vi "Aero_tunnel_monitor_on_OGI.vi"() -> ()   [LabVIEW 2014]
uses:
  Controls/Post_Process.ctl
  <vilib>/Platform/TimedLoop/XDataNode/timing_clust.ctl
  <vilib>/Platform/TimedLoop/XDataNode/nitl_modes.ctl
  <vilib>/Platform/TimedLoop/XDataNode/wakeup.ctl
  ADAM Client/Sub VIs/ADAM Controls/Update_scan_value.ctl
  Globals/Meas_global.vi
  <vilib>/Platform/TimedLoop/XDataNode/XDataNode.xnode
  <vilib>/Platform/TimedLoop/XDataNode/XDNodeRunTimeDep.lvlib
panel:
  in  "Use Polynomial for Ratio":bool
  in  "Manual Ratio":dbl=1.02
  in  "Display Graph?":bool
  in  "Menu Ring":u16(ring) items=["Lift", "Pitch", "Drag", "Side", "Yaw", "Roll"]
  in  "Samples":i32=1000
  out "Waveform Chart":dbl[](graph)
  in  "Output Roll":bool
  out "Roll":string="0.0 Nm"
  in  "Output Yaw":bool
  out "Yaw":string="0.0 Nm"
  in  "Output Pitch":bool
  out "Pitch":string="0.0 Nm"
  in  "Output SF":bool
  out "SF":string="0.0 N"
  in  "Output Drag":bool
  out "Drag":string="0.0 N"
  in  "Output Lift":bool
  out "Lift":string="0.0 N"
  in  "Balance Safety limits":T1(array[cluster])=[{"Max +ve Range"=80, "Max -ve Range"=80, "Axis"="Lift"}, {"Max +ve Range"=80, "Max -ve Range"=80, "Axis"="Pitch"}, {"Max +ve Range"=80, "Max -ve Range"=80, "Axis"="Drag"}, {"Max +ve Range"=80, "Max -ve Range"=80, "Axis"="Side-Force"}, {"Max +ve Range"=99, "Max -ve Range"=99, "Axis"="Yaw"}, {"Max +ve Range"=80, "Max -ve Range"=80, "Axis"="Roll"}] {"Max -ve Range" min=0 max=125; "Max +ve Range" min=0 max=125}
  out "Monitor Speed (Hz)":dbl
  out "Belt slip warning":bool
  out "Road Status":string="???"
  in  "GotoYaw":bool
  in  "NewYawPos":dbl
  out "YAW POSITION":dbl
  out "Required WindSpeedRatio":dbl
  out "ROAD SPEED m/s":dbl
  in  "BL Fan1":i32
  in  "BL Fan2":i32
  in  "Stop drive":bool
  in  "Start Drive":bool
  in  "Synch to Wind":bool
  out "Road Info":string="???"
  in  "stop":bool
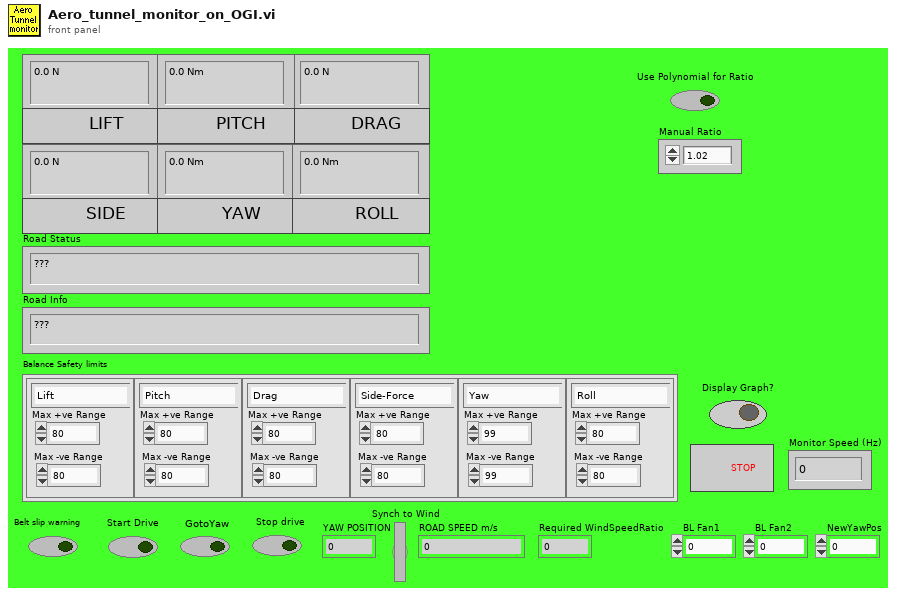
[diagram p1: front panel]
types:
  T1 = cluster{"Max +ve Range":i32, "Max -ve Range":i32, "Axis":string}[]
  T2 = typedef "Post_Process.ctl" = enum16{"Take New Data", "Post Process Raw Data File"}
  T3 = typedef "XDNodeRunTimeDep.lvlib/timing_clust.ctl" = cluster{"Expected End [f-1]":u64, "Actual End [f-1]":u64, "Finished Late? [f-1]":bool, "Expected End [i-1]":u64, "Actual End [i-1]":u64, "Finished Late? [i-1]":bool, "Expected Start [i]":u64, "Actual Start [i]":u64, "Expected Start [f]":u64, "Actual Start [f]":u64, "Source Name":string, "Structure Name":string, "Period":i64, "Deadline":i64, "Offset":i64, "Start":i64, "Priority":i32, "Timeout":i32, "Mode":T4, "Wakeup Reason":T5, "Error":errorcluster, "Source Type":string, "Secondary Source Type":string, "Global End Time":u64, "Global Start Time":u64, "Frame Duration":u64, "Iteration Duration":u64, "Assigned CPU":i32, "I/O Scan Engine Mode":u32}
  T4 = typedef "XDNodeRunTimeDep.lvlib/nitl_modes.ctl" = enum32{"No Change", "Process missed periods, maintain original phase", "Discard missed periods, maintain original phase", "Process missed periods, ignore original phase", "Discard missed periods, ignore original phase"}
  T5 = typedef "XDNodeRunTimeDep.lvlib/wakeup.ctl" = enum32{"Normal", "Aborted", "Asynchronous wakeup", "Timing source error", "Timed loop error", "Timeout"}
  T6 = typedef "Update_scan_value.ctl" = cluster{"Channel Name":string, "New Value":dbl}
  T7 = cluster{"Max +ve Range":i32, "Max -ve Range":i32, "Axis":string}
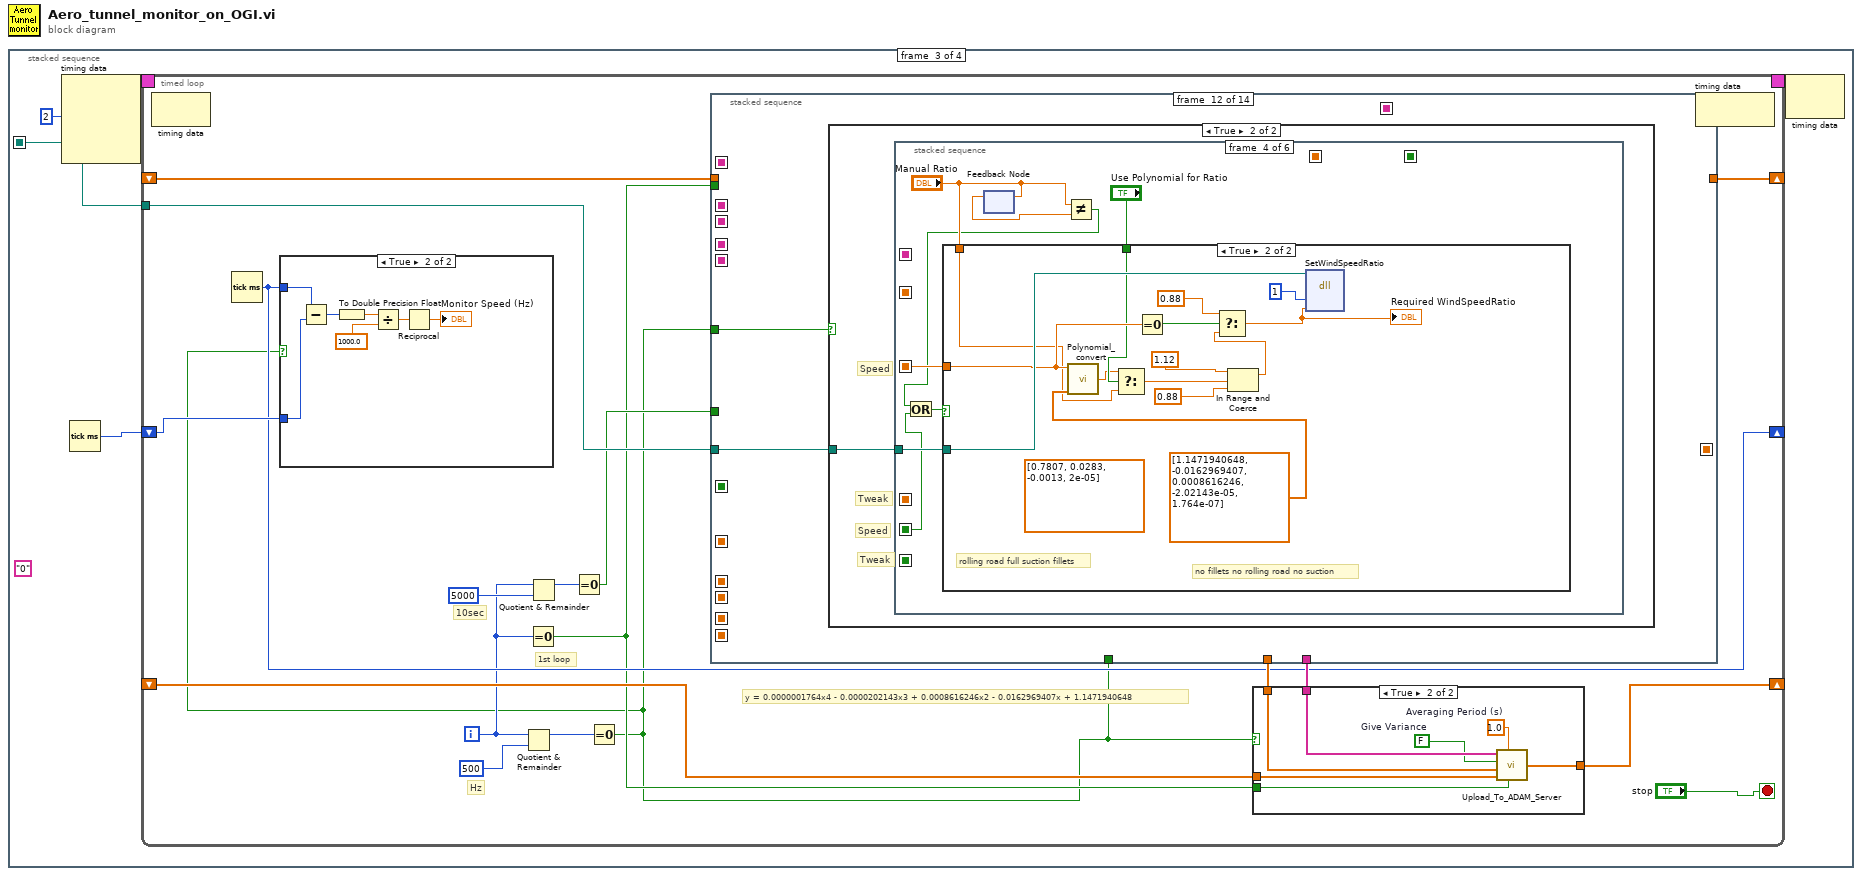
[diagram p0: block diagram]
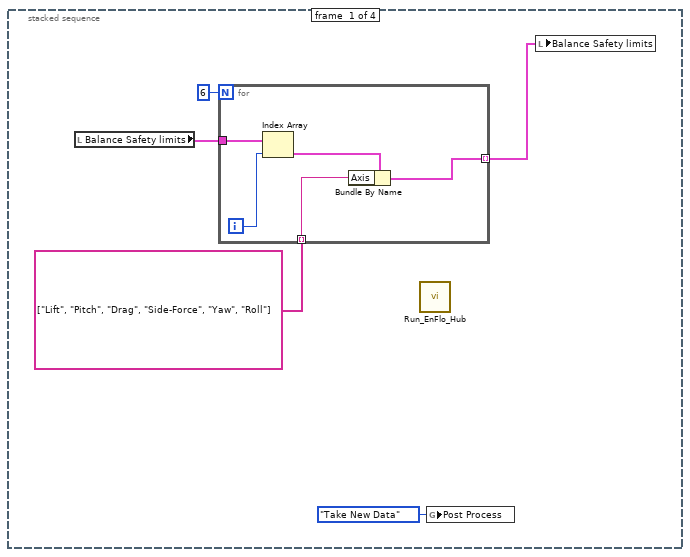
[diagram p2: hidden frame]
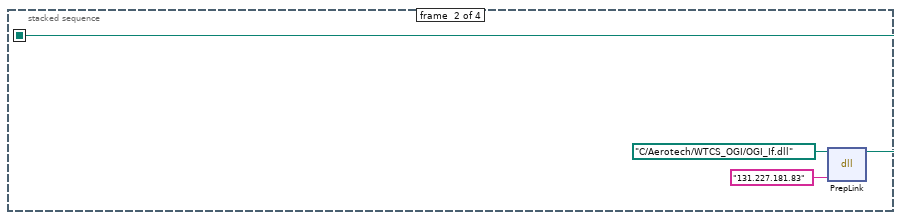
[diagram p3: hidden frame]
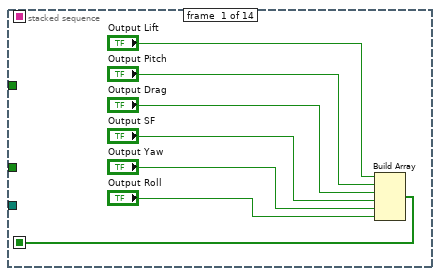
[diagram p6: hidden frame]
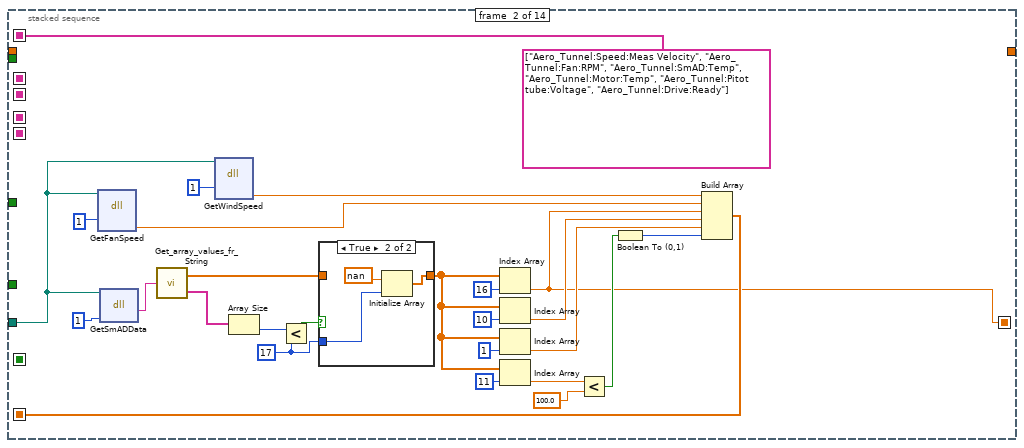
[diagram p7: hidden frame]
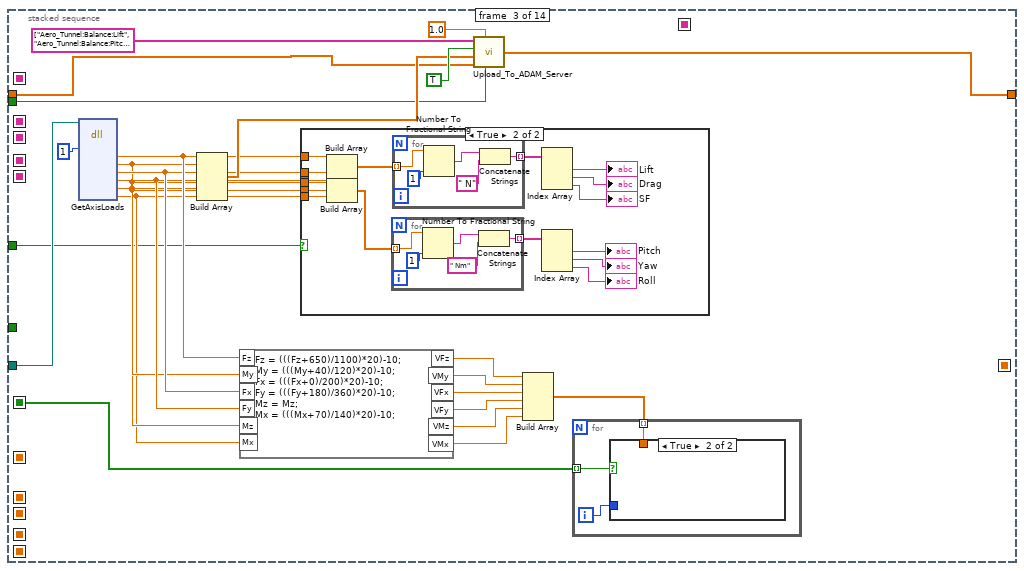
[diagram p9: hidden frame]
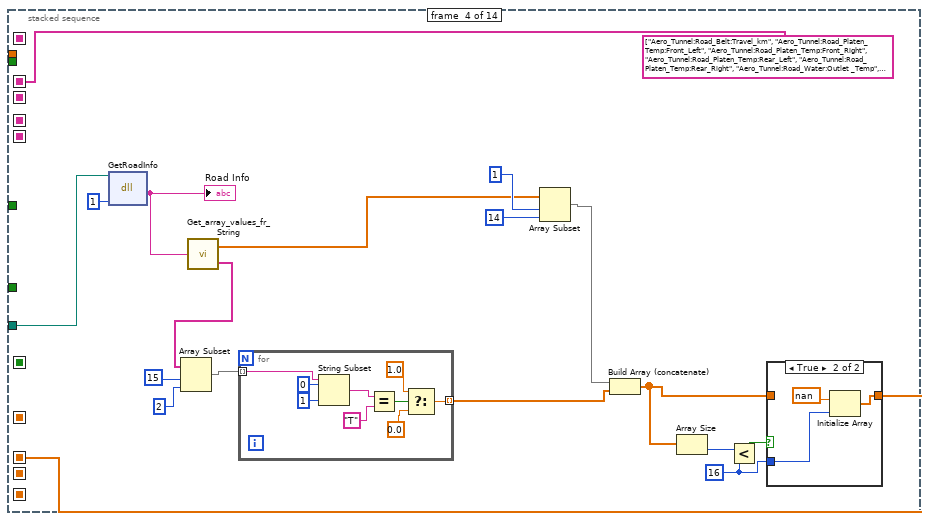
[diagram p12: hidden frame]
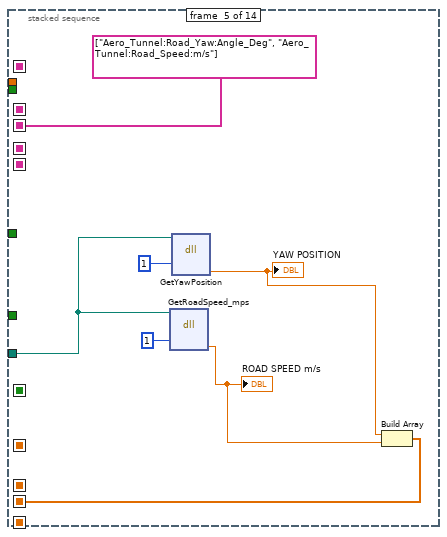
[diagram p14: hidden frame]
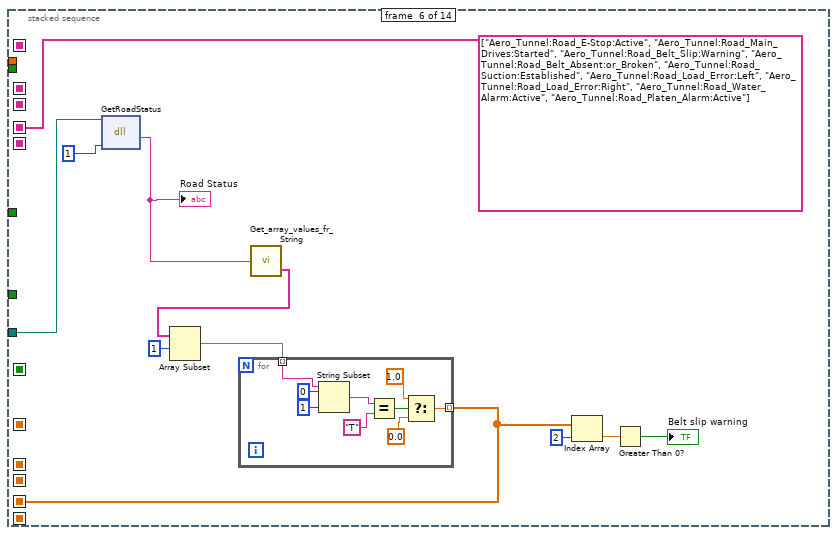
[diagram p15: hidden frame]
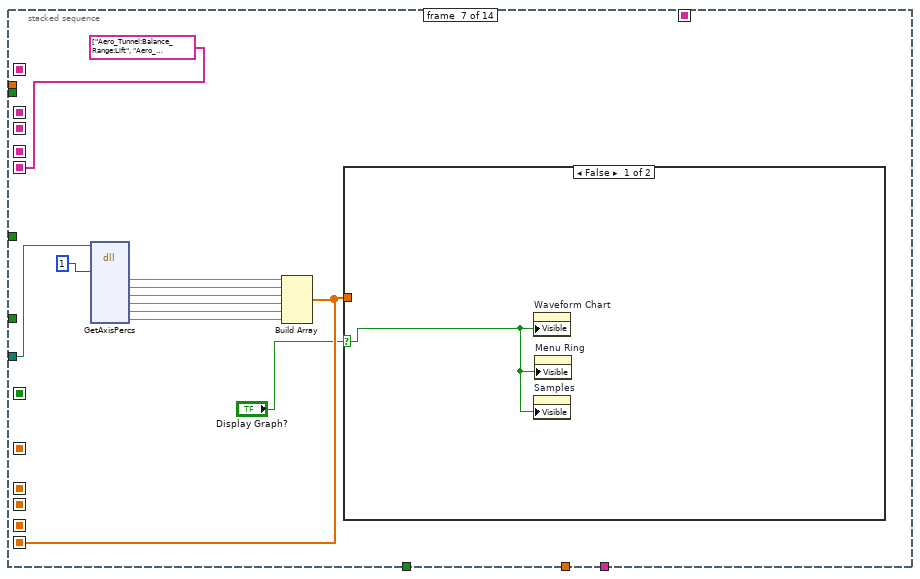
[diagram p16: hidden frame]
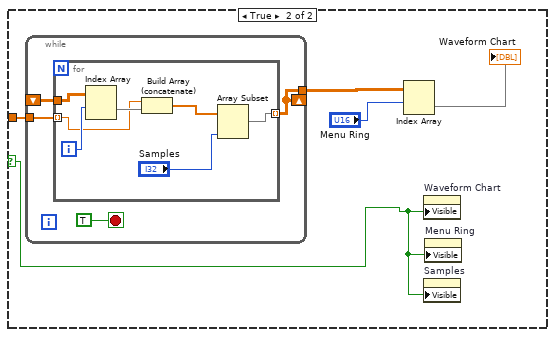
[diagram p17: hidden frame]
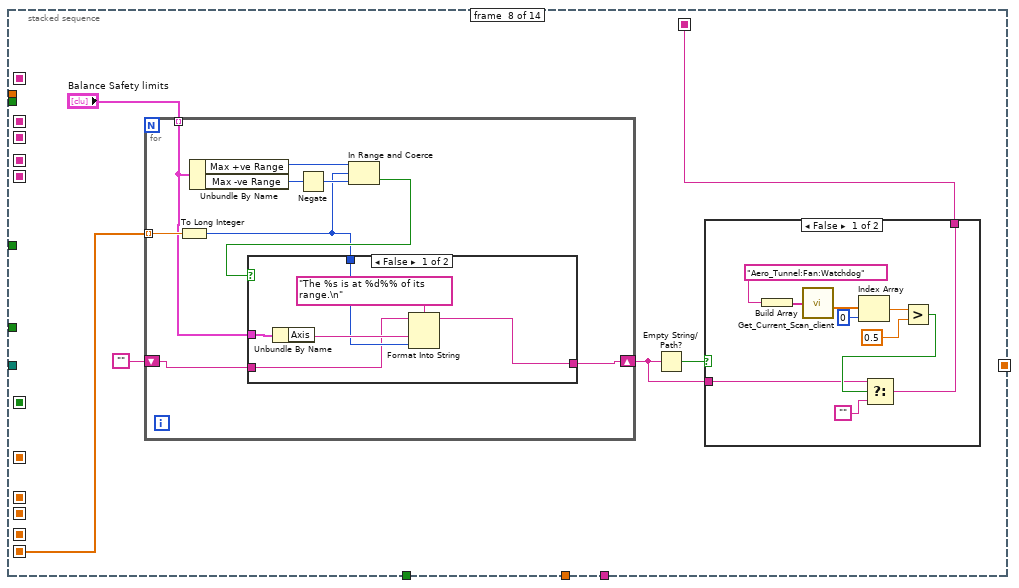
[diagram p18: hidden frame]
diagram:
  n1 = stacked-sequence {
    seq-local: [_ w11 _ _] -> [_ _ w18 w513]
    frame #0 {
      n2 = local read "Balance Safety limits"() -> (w4:T1)
      n3 = for {
        N: 6 -> [_]
        tunnel: w4 -> [w10]
        tunnel: [w7] -> w3 mode=indexing
        tunnel: string[] ["Lift", "Pitch", "Drag", "Side-Force", "Yaw", "Roll"] ("Channel Names") -> [w6] mode=indexing
        i -> [w9]
        n4 = Index Array(array=w10, index=w9) -> (element=w8:T7)
        n5 = Bundle By Name(cluster=w8, "Axis"=w6) -> (w7:T7)
      }
      n6 = call "Run_EnFlo_Hub.vi"() -> ()  [unwired: 8 in]
      n7 = global write "Meas_global.vi" "Post Process"(Post_Process."Take New Data" ("Post Process")) -> ()
      n8 = local write "Balance Safety limits"(w3) -> ()
    }
    frame #1 {
      n9 = dll-call lib="C:/Aerotech/Drivers/OGI_IF.dll" fn="PrepLink"(path in=path "C:/Aerotech/WTCS_OGI/OGI_If.dll", "IPAddress"="131.227.181.83") -> (path out=w11:path)  [unwired: 2 in, 3 out]
    }
    frame #2 {
      (unwired) "0" ("Channels")
      n10 = node-c288(i64 2 ("Period")) -> (w16:T3)  [unwired: 3 in]
      n11 = Tick Count (ms)() -> (millisecond timer value=w17:u32)
      n12 = timed-loop {
        shift-right: [w36] -> _
        shift-left: _ -> [w34]
        tunnel: w18 -> [w32]
        shift-right: [w30] -> _
        shift-left: _ -> [w31]
        timing: w16 -> [_]
        timing-out: [_] -> w15
        shift-right: [w28] -> _
        shift-left: w17 -> [w29]
        i -> [w22]
        stop <- "stop" stop-if-true
        # "1st loop"
        # "10sec"
        # "Hz"
        # "y = 0.0000001764x4 - 0.0000202143x3 + 0.0008616246x2 - 0.0162969407x + 1.1471940648"
        n13 = node-c288() -> ()  [unwired: 1 in, 1 out]
        n14 = Tick Count (ms)() -> (millisecond timer value=w28:u32)
        n15 = Quotient & Remainder(x=w22, y=500) -> (x-y*floor(x/y)=w25:i32)  [unwired: 1 out]
        n16 = Equal To 0?(x=w22) -> (x = 0?=w21:bool)
        n17 = Quotient & Remainder(x=w22, y=5000) -> (x-y*floor(x/y)=w24:i32)  [unwired: 1 out]
        n18 = Equal To 0?(x=w24) -> (x = 0?=w23:bool)
        n19 = Equal To 0?(x=w25) -> (x = 0?=w20:bool)
        n20 = case shown="True" w20 {
          tunnel: w29 -> [_ w43]
          tunnel: w28 -> [_ w42]
          frame False {
          }
          frame True {
            n21 = Subtract(x=w42, y=w43) -> (x-y=w41:u32)
            n22 = To Double Precision Float(number=w41) -> (double precision float=w37:dbl)
            n23 = Divide(x=w37, y=1000.0) -> (x/y=w39:dbl)
            n24 = Reciprocal(x=w39) -> (1/x=→"Monitor Speed (Hz)":dbl)
          }
        }
        n25 = stacked-sequence {
          seq-local: [_ string[] ["Aero_Tunnel:Speed:Meas Velocity", "Aero_Tunnel:Fan:RPM", "Aero_Tunnel:SmAD:Temp", "Aero_Tunnel:Motor:Temp", "Aero_Tunnel:Pitot tube:Voltage", "Aero_Tunnel:Drive:Ready"] ("Channel Names") _ _ _ _ _ _ _ _ _ _ _ _] -> [_ _ _ _ _ _ _ _ _ _ w319 _ _ _]
          seq-local: [_ w76 _ _ _ _ _ _ _ _ _ _ _ _] -> [_ _ _ _ _ _ _ _ _ _ w318 _ _ _]
          seq-local: [_ _ _ w144 _ _ _ _ _ _ _ _ _ _] -> [_ _ _ _ _ _ _ _ _ _ w315 _ _ _]
          seq-local: [_ _ _ string[] ["Aero_Tunnel:Road_Belt:Travel_km", "Aero_Tunnel:Road_Platen_Temp:Front_Left", "Aero_Tunnel:Road_Platen_Temp:Front_Right", "Aero_Tunnel:Road_Platen_Temp:Rear_Left", "Aero_Tunnel:Road_Platen_Temp:Rear_Right", "Aero_Tunnel:Road_Water:Outlet _Temp", "Aero_Tunnel:Road_Water:Inlet _Temp", "Aero_Tunnel:Road_Suction:Front", "Aero_Tunnel:Road_Suction:Middle", "Aero_Tunnel:Road_Suction:Rear", "Aero_Tunnel:Road_BL_Suction:Primary", "Aero_Tunnel:Road_BL_Suction:Secondary", "Aero_Tunnel:Road_LoadCell:Left", "Aero_Tunnel:Road_LoadCell:Right", "Aero_Tunnel:Road_Water_High:Temp_Alarm", "Aero_Tunnel:Road_Platen_High:Temp_Alarm"] ("Channel Names") _ _ _ _ _ _ _ _ _ _] -> [_ _ _ _ _ _ _ _ _ _ w304 _ _ _]
          seq-local: [_ _ _ _ string[] ["Aero_Tunnel:Road_Yaw:Angle_Deg", "Aero_Tunnel:Road_Speed:m/s"] ("Channel Names") _ _ _ _ _ _ _ _ _] -> [_ _ _ _ _ _ _ _ _ _ w314 _ _ _]
          seq-local: [_ _ _ _ w175 _ _ _ _ _ _ _ _ _] -> [_ _ _ _ _ _ _ _ _ _ w313 _ _ _]
          seq-local: [_ _ _ _ _ string[] ["Aero_Tunnel:Road_E-Stop:Active", "Aero_Tunnel:Road_Main_Drives:Started", "Aero_Tunnel:Road_Belt_Slip:Warning", "Aero_Tunnel:Road_Belt_Absent:or_Broken", "Aero_Tunnel:Road_Suction:Established", "Aero_Tunnel:Road_Load_Error:Left", "Aero_Tunnel:Road_Load_Error:Right", "Aero_Tunnel:Road_Water_Alarm:Active", "Aero_Tunnel:Road_Platen_Alarm:Active"] ("Channel Names") _ _ _ _ _ _ _ _] -> [_ _ _ _ _ _ _ _ _ _ w309 _ _ _]
          seq-local: [_ _ _ _ _ w188 _ _ _ _ _ _ _ _] -> [_ _ _ _ _ _ _ _ _ _ w308 _ _ _]
          seq-local: [w54 _ _ _ _ _ _ _ _ _ _ _ _ _] -> [_ _ w106 _ _ _ _ _ _ _ _ _ _ _]
          seq-local: [_ _ _ _ _ _ string[] ["Aero_Tunnel:Balance_Range:Lift", "Aero_Tunnel:Balance_Range:Pitch", "Aero_Tunnel:Balance_Range:Drag", "Aero_Tunnel:Balance_Range:Side-Force", "Aero_Tunnel:Balance_Range:Yaw", "Aero_Tunnel:Balance_Range:Roll"] ("Channel Names") _ _ _ _ _ _ _] -> [_ _ _ _ _ _ _ _ _ _ w305 _ _ _]
          seq-local: [_ _ _ _ _ _ w203 _ _ _ _ _ _ _] -> [_ _ _ _ _ _ _ w234 _ _ w306 _ _ _]
          seq-local: [_ _ _ _ _ _ _ w230 _ _ _ _ _ _] -> [_ _ _ _ _ _ _ _ w264 w283 _ _ _ _]
          seq-local: [_ w61 _ _ _ _ _ _ _ _ _ _ _ _] -> [_ _ _ _ _ _ _ _ _ w282 _ _ _ _]
          tunnel: [_ _ _ _ _ _ _ _ _ _ w317 _ _ _] -> w35
          tunnel: [_ _ _ _ _ _ _ _ _ _ w316 _ _ _] -> w33
          tunnel: w32 -> [_ w68 w113 w160 w178 w191 w212 _ _ _ w307 w321 w416 w443]
          tunnel: w20 -> [_ _ _ _ _ _ _ _ _ _ _ _ _ _]
          tunnel: w31 -> [_ _ w100 _ _ _ _ _ _ _ _ _ _ _]
          tunnel: [_ _ w99 _ _ _ _ _ _ _ _ _ _ _] -> w30
          tunnel: w20 -> [_ _ w92 _ _ _ _ _ _ _ _ w320 _ w442]
          tunnel: w23 -> [_ _ _ _ _ _ _ _ w263 _ _ _ w415 _]
          tunnel: w21 -> [_ _ w91 _ _ _ _ _ _ _ _ _ _ _]
          frame #0 {
            n26 = Build Array("Output Lift", "Output Pitch", "Output Drag", "Output SF", "Output Yaw", "Output Roll") -> (w54:bool[])
          }
          frame #1 {
            w62 = 17 ("y")
            n27 = dll-call lib="C:/Aerotech/Drivers/OGI_IF.dll" fn="GetFanSpeed"(path in=w68, "Enable"=1) -> ("FanSpeedinRPM"=w70:dbl)  [unwired: 3 in, 4 out]
            n28 = dll-call lib="C:/Aerotech/Drivers/OGI_IF.dll" fn="GetSmADData"(path in=w68, "Enable"=1) -> ("SmAD Data String"=w73:string)  [unwired: 2 in, 3 out]
            n29 = call "Get_array_values_fr_String.vi"("String Value"=w73) -> ("Numeric Array"=w63:dbl[], "String array"=w66:string[])
            n30 = dll-call lib="C:/Aerotech/Drivers/OGI_IF.dll" fn="GetWindSpeed"(path in=w68, "Enable"=1) -> ("Windspeed_M/s"=w69:dbl)  [unwired: 3 in, 4 out]
            n31 = Array Size(array=w66) -> (size(s)=w67:i32)
            n32 = Less?(x=w67, y=w62) -> (x < y?=w65:bool)
            n33 = case shown="True" w65 {
              tunnel: [w87 w90] -> w64
              tunnel: w63 -> [w87 _]
              tunnel: w62 -> [_ w88]
              frame False {
              }
              frame True {
                n34 = Initialize Array(nan, w88) -> (w90:dbl[])
              }
            }
            n35 = Index Array(array=w64, index=16) -> (element=w61:dbl)
            n36 = Index Array(array=w64, index=10) -> (element=w84:dbl)
            n37 = Index Array(array=w64, index=1) -> (element=w82:dbl)
            n38 = Index Array(array=w64, index=11) -> (element=w80:dbl)
            n39 = Less?(x=w80, y=100.0) -> (x < y?=w78:bool)
            n40 = Boolean To (0,1)(Boolean=w78) -> (0, 1=w77:i16)
            n41 = Build Array(w69, w70, w61, w84, w82, w77) -> (w76:dbl[])
          }
          frame #2 {
            n42 = dll-call lib="C:/Aerotech/Drivers/OGI_IF.dll" fn="GetAxisLoads"(path in=w113, "Enable"=1) -> ("Lift"=w98:dbl, "Pitch"=w95:dbl, "Drag"=w97:dbl, "side"=w96:dbl, "Yaw"=w94:dbl, "Roll"=w93:dbl)  [unwired: 3 in, 9 out]
            n43 = Build Array(w98, w95, w97, w96, w94, w93) -> (w101:dbl[])
            n44 = formula code="VFz = (((Fz+650)/1100)*20)-10;\nVMy = (((My+40)/120)*20)-10;\nVFx = (((Fx+0)/200)*20)-10;\nVFy = (((Fy+180)/360)*20)-10;\nVMz = Mz;\nVMx = (((Mx+70)/140)*20)-10;"("Fz"=w98, "My"=w95, "Fx"=w97, "Fy"=w96, "Mz"=w94, "Mx"=w93) -> ("VFz"=w112:dbl, "VMy"=w111:dbl, "VFx"=w110:dbl, "VFy"=w109:dbl, "VMz"=w108:dbl, "VMx"=w107:dbl)
            n45 = case shown="True" w92 {
              tunnel: w98 -> [_ w130]
              tunnel: w97 -> [_ w129]
              tunnel: w96 -> [_ w128]
              tunnel: w95 -> [_ w122]
              tunnel: w94 -> [_ w121]
              tunnel: w93 -> [_ w120]
              frame False {
              }
              frame True {
                n46 = Build Array(w130, w129, w128) -> (w127:dbl[])
                n47 = Build Array(w122, w121, w120) -> (w119:dbl[])
                n48 = for {
                  tunnel: w119 -> [w131] mode=indexing
                  tunnel: [w135] -> w118 mode=indexing
                  n49 = Number To Fractional String(number=w131, precision (6)=i16 1) -> (F-format string=w132:string)  [unwired: 2 in]
                  n50 = Concatenate Strings(w132, " Nm" ("string")) -> (w135:string)
                }
                n51 = for {
                  tunnel: w127 -> [w136] mode=indexing
                  tunnel: [w140] -> w126 mode=indexing
                  n52 = Number To Fractional String(number=w136, precision (6)=i16 1) -> (F-format string=w137:string)  [unwired: 2 in]
                  n53 = Concatenate Strings(w137, " N" ("string")) -> (w140:string)
                }
                n54 = Index Array(array=w126) -> (element #1=→"Lift":string, element #2=→"Drag":string, element #3=→"SF":string)  [unwired: 3 in]
                n55 = Index Array(array=w118) -> (element #1=→"Pitch":string, element #2=→"Yaw":string, element #3=→"Roll":string)  [unwired: 3 in]
              }
            }
            n56 = call "Upload_To_ADAM_Server.vi"("First Loop"=w91, "Averaging Period (s)"=1.0, "Shift In"=w100, "Channel Values"=w101, "Give Variance"=TRUE, "Channel Names"=string[] ["Aero_Tunnel:Balance:Lift", "Aero_Tunnel:Balance:Pitch", "Aero_Tunnel:Balance:Drag", "Aero_Tunnel:Balance:Side-Force", "Aero_Tunnel:Balance:Yaw", "Aero_Tunnel:Balance:Roll"]) -> ("Shift Out"=w99:dbl[])
            n57 = Build Array(w112, w111, w110, w109, w108, w107) -> (w105:dbl[])
            n58 = for {
              tunnel: w106 -> [w143] mode=indexing
              tunnel: w105 -> [w142] mode=indexing
              i -> [w141]
              n59 = case shown="True" w143 {
                tunnel: w142 -> [_ _]
                tunnel: w141 -> [_ _]
                frame False {
                }
                frame True {
                }
              }
            }
          }
          frame #3 {
            w147 = 16 ("y")
            n60 = dll-call lib="C:/Aerotech/Drivers/OGI_IF.dll" fn="GetRoadInfo"(path in=w160, "Enable"=1) -> ("Road Info"=w159:string)  [unwired: 3 in, 2 out]
            "Road Info" <- w159
            n61 = call "Get_array_values_fr_String.vi"("String Value"=w159) -> ("Numeric Array"=w146:dbl[], "String array"=w150:string[])
            n62 = Array Subset(array=w150, index=15, length=2) -> (w154:string[])
            n63 = for {
              tunnel: w154 -> [w172] mode=indexing
              tunnel: [w166] -> w153 mode=indexing
              n64 = String Subset(string=w172, offset (0)=0, length (rest)=1 ("length (rest)")) -> (substring=w171:string)
              n65 = Equal?(x=w171, y="T") -> (x = y?=w169:bool)
              n66 = Select(t=1.0, s=w169, f=0.0) -> (s? t:f=w166:dbl)
            }
            n67 = Array Subset(array=w146, index=1, length=14) -> (w152:dbl[])
            n68 = Build Array (concatenate)(w152, w153) -> (w145:dbl[])
            n69 = Array Size(array=w145) -> (size(s)=w149:i32)
            n70 = Less?(x=w149, y=w147) -> (x < y?=w148:bool)
            n71 = case shown="True" w148 {
              tunnel: [w162 w165] -> w144
              tunnel: w145 -> [w162 _]
              tunnel: w147 -> [_ w163]
              frame False {
              }
              frame True {
                n72 = Initialize Array(nan, w163) -> (w165:dbl[])
              }
            }
          }
          frame #4 {
            n73 = dll-call lib="C:/Aerotech/Drivers/OGI_IF.dll" fn="GetRoadSpeed_mps"(path in=w178, "Enable"=1) -> ("RoadSpeed_mps"=w176:dbl)  [unwired: 3 in, 4 out]
            "ROAD SPEED m/s" <- w176
            n74 = dll-call lib="C:/Aerotech/Drivers/OGI_IF.dll" fn="GetYawPosition"(path in=w178, "Enable"=1) -> ("Yaw Position"=w177:dbl)  [unwired: 3 in, 4 out]
            "YAW POSITION" <- w177
            n75 = Build Array(w177, w176) -> (w175:dbl[])
          }
          frame #5 {
            n76 = dll-call lib="C:/Aerotech/Drivers/OGI_IF.dll" fn="GetRoadStatus"(path in=w191, "Enable"=1) -> ("Road Status"=w190:string)  [unwired: 3 in, 2 out]
            "Road Status" <- w190
            n77 = call "Get_array_values_fr_String.vi"("String Value"=w190) -> ("String array"=w184:string[])  [unwired: 1 out]
            n78 = Array Subset(array=w184, index=1) -> (w182:string[])  [unwired: 1 in]
            n79 = for {
              tunnel: [w194] -> w188 mode=indexing
              tunnel: w182 -> [w193] mode=indexing
              n80 = String Subset(string=w193, offset (0)=0, length (rest)=1 ("length (rest)")) -> (substring=w199:string)
              n81 = Equal?(x=w199, y="T") -> (x = y?=w197:bool)
              n82 = Select(t=1.0, s=w197, f=0.0) -> (s? t:f=w194:dbl)
            }
            n83 = Index Array(array=w188, index=2) -> (element=w186:dbl)
            n84 = Greater Than 0?(x=w186) -> (x > 0?=→"Belt slip warning":bool)
          }
          frame #6 {
            n85 = dll-call lib="C:/Aerotech/Drivers/OGI_IF.dll" fn="GetAxisPercs"(path in=w212, "Enable"=1) -> ("Lift"=w210:dbl, "Pitch"=w209:dbl, "Drag"=w208:dbl, "side"=w207:dbl, "Yaw"=w206:dbl, "Roll"=w205:dbl)  [unwired: 3 in, 9 out]
            n86 = Build Array(w210, w209, w208, w207, w206, w205) -> (w203:dbl[])
            n87 = case shown="False" "Display Graph?" {
              selector: "Display Graph?" -> [w213 w214]
              tunnel: w203 -> [_ w218]
              frame False {
                n88 = property on="Waveform Chart" class="WFChart (strict)"("Visible"=w213) -> ()  [unwired: 2 in, 2 out]
                n89 = property on="Samples" class="DigNum (strict)"("Visible"=w213) -> ()  [unwired: 2 in, 2 out]
                n90 = property on="Menu Ring" class="Ring (strict)"("Visible"=w213) -> ()  [unwired: 2 in, 2 out]
              }
              frame True {
                n91 = while {
                  shift-right: [w220] -> _
                  shift-left: _ -> [w222]
                  tunnel: w218 -> [w221]
                  tunnel: [w220] -> w217
                  stop <- TRUE stop-if-true
                  n92 = for {
                    tunnel: w222 -> [w225]
                    tunnel: w221 -> [w223] mode=indexing
                    tunnel: [w228] -> w220 mode=indexing
                    i -> [w226]
                    n93 = Index Array(array=w225, index (row)=w226) -> (element=w224:dbl[])  [unwired: 1 in]
                    n94 = Build Array (concatenate)(w223, w224) -> (w229:dbl[])
                    n95 = Array Subset(array=w229, length="Samples") -> (w228:dbl[])  [unwired: 1 in]
                  }
                }
                n96 = Index Array(array=w217, index (row)="Menu Ring") -> (element=→"Waveform Chart":dbl[])  [unwired: 1 in]
                n97 = property on="Waveform Chart" class="WFChart (strict)"("Visible"=w214) -> ()  [unwired: 2 in, 2 out]
                n98 = property on="Samples" class="DigNum (strict)"("Visible"=w214) -> ()  [unwired: 2 in, 2 out]
                n99 = property on="Menu Ring" class="Ring (strict)"("Visible"=w214) -> ()  [unwired: 2 in, 2 out]
              }
            }
          }
          frame #7 {
            n100 = for {
              tunnel: "Balance Safety limits" -> [w250] mode=indexing
              tunnel: w234 -> [w253] mode=indexing
              shift-right: [w247] -> w231
              shift-left: "" -> [w248]
              n101 = To Long Integer(number=w253) -> (32bit integer=w249:i32)
              n102 = Unbundle By Name(w250) -> ("Max +ve Range"=w255:i32, "Max -ve Range"=w254:i32)
              n103 = Negate(x=w254) -> (-x=w252:i32)
              n104 = In Range and Coerce(upper limit=w255, x=w249, lower limit=w252) -> (In Range?=w251:bool)  [unwired: 1 out]
              n105 = case shown="False" w251 {
                tunnel: w250 -> [w261 _]
                tunnel: w249 -> [w259 _]
                tunnel: w248 -> [w257 w262]
                tunnel: [w256 w262] -> w247
                frame False {
                  n106 = Unbundle By Name(w261) -> ("Axis"=w260:string)
                  n107 = Format Into String(format string="The %s is at %d%% of its range.\n", initial string=w257, w260, w259) -> (resulting string=w256:string)  [unwired: 1 in, 1 out]
                }
                frame True {
                }
              }
            }
            n108 = Empty String/Path?(string/path=w231) -> (empty?=w232:bool)
            n109 = case shown="False" w232 {
              tunnel: w231 -> [w238 w246]
              tunnel: [w236 w246] -> w230
              frame False {
                n110 = Build Array("Aero_Tunnel:Fan:Watchdog") -> (w245:string[])
                n111 = call "Get_Current_Scan_client.vi"("ADAM Ch Names"=w245) -> ("Numerical Values"=w243:dbl[])  [unwired: 1 in, 2 out]
                n112 = Index Array(array=w243, index=0) -> (element=w241:dbl)
                n113 = Greater?(x=w241, y=0.5) -> (0:w239:bool)
                n114 = Select(t=w238, s=w239, f="") -> (s? t:f=w236:string)
              }
              frame True {
              }
            }
          }
          frame #8 {
            n115 = while {
              tunnel: w264 -> [w268]
              tunnel: w263 -> [w265]
              stop <- TRUE stop-if-true
              n116 = Empty String/Path?(string/path=w268) -> (empty?=w270:bool)
              n117 = Not(x=w270) -> (.not. x?=w266:bool)
              n118 = Compound Arithmetic op=AND(w266, w265) -> (w269:bool)
              n119 = case shown="True" w269 {
                tunnel: w268 -> [_ w275]
                frame False {
                }
                frame True {
                  w274 = string[] ["Aero_Tunnel:Fan:Watchdog", "Aero_Tunnel:Road:Watchdog", "Aero_Tunnel:Speed:Dem Velocity"] ("Channel Names")
                  n120 = Format Into String(format string="The Aero Tunnel balance has gone outside of its limits.\n%s\nThe Aero_Tunnel:Fan:Watchdog has therefore been disabled. ", w275) -> (resulting string=w276:string)  [unwired: 2 in, 1 out]
                  n121 = Bundle By Name(cluster=errorcluster {"status"=TRUE, "code"=0, "source"=""} ("error in (no error)"), "source"=w276) -> (w278:errorcluster)
                  n122 = Array Size(array=w274) -> (size(s)=w273:i32)
                  n123 = call "EnFlo_Error_Handler.vi"("error in (no error)"=w278, "Error Type"="Aero Tunnel Balance Range Trip", "Dialog Box (T)"=FALSE) -> ()  [unwired: 3 out]
                  n124 = Initialize Array(0.0, w273) -> (w271:dbl[])
                  n125 = call "ASYNC_Adam_client.vi"("Values"=w271, "Channel Names"=w274) -> ()  [unwired: 1 in, 2 out]
                }
              }
            }
          }
          frame #9 {
            n126 = while {
              tunnel: w283 -> [_]
              shift-right: [w288] -> _
              shift-left: _ -> [w287]
              tunnel: w282 -> [w285]
              stop <- TRUE stop-if-true
              n127 = Greater?(x=w285, y=35.0) -> (0:w288:bool)
              n128 = Number To Fractional String(number=w285, precision (6)=i16 2) -> (F-format string=w284:string)  [unwired: 2 in]
              n129 = Compound Arithmetic op=AND(invert w287, w288) -> (w291:bool)
              n130 = case shown="True" w291 {
                tunnel: w284 -> [_ w296]
                frame False {
                }
                frame True {
                  w295 = string[] ["Aero_Tunnel:Fan:Watchdog", "Aero_Tunnel:Road:Watchdog", "Aero_Tunnel:Speed:Dem Velocity"] ("Channel Names")
                  n131 = Format Into String(format string="The Aero Tunnel temperature has gone above it's limits and is:\n%s\nThe Aero_Tunnel:Fan:Watchdog has therefore been disabled. ", w296) -> (resulting string=w297:string)  [unwired: 2 in, 1 out]
                  n132 = Bundle By Name(cluster=errorcluster {"status"=TRUE, "code"=0, "source"=""} ("error in (no error)"), "source"=w297) -> (w299:errorcluster)
                  n133 = Array Size(array=w295) -> (size(s)=w294:i32)
                  n134 = call "EnFlo_Error_Handler.vi"("error in (no error)"=w299, "Error Type"="Aero Tunnel Temperature Trip", "Dialog Box (T)"=FALSE) -> ()  [unwired: 3 out]
                  n135 = Initialize Array(0.0, w294) -> (w292:dbl[])
                  n136 = call "ASYNC_Adam_client.vi"("Values"=w292, "Channel Names"=w295) -> ()  [unwired: 1 in, 2 out]
                }
              }
            }
          }
          frame #10 {
            n137 = Build Array (concatenate)(w318, w315, w313, w308, w306) -> (w317:dbl[])
            n138 = Boolean To (0,1)(Boolean="GotoYaw") -> (0, 1=w312:i16)
            n139 = Build Array (concatenate)(w319, w304, w314, w309, w305) -> (w316:string[])
            n140 = To Long Integer(number=w312) -> (32bit integer=w303:i32)
            n141 = dll-call lib="C:/Aerotech/Drivers/OGI_IF.dll" fn="GotoYawPosition"(path in=w307, "Enable"=w303, "NewYawPos"="NewYawPos") -> ()  [unwired: 3 in, 4 out]
          }
          frame #11 {
            n142 = case shown="True" w320 {
              tunnel: w321 -> [_ w322]
              frame False {
              }
              frame True {
                # "Tweak"
                # "Speed"
                # "Tweak"
                # "Speed"
                n143 = stacked-sequence {
                  seq-local: [_ w336 _ _ _ _] -> [_ _ _ w381 _ _]
                  seq-local: [_ w327 _ _ _ _] -> [_ _ _ w377 _ _]
                  seq-local: [_ w334 _ _ _ _] -> [_ _ _ _ w397 _]
                  seq-local: [_ w330 _ _ _ _] -> [_ _ _ _ _ w406]
                  seq-local: [_ w328 _ _ _ _] -> [_ _ _ _ _ _]
                  seq-local: [_ w326 _ _ _ _] -> [_ _ _ _ _ _]
                  seq-local: [string[] ["Aero_Tunnel:Speed:Dem Velocity", "Froude:NPL:Atmos_Press", "Aero_Tunnel:Motor:Enable", "Aero_Tunnel:Speed:Calib Tweak", "Aero_Tunnel:Upper:Temp", "Aero_Tunnel:Lower:Temp", "Aero_Tunnel:Fan:Watchdog"] ("appended array") _ _ _ _ _] -> [_ w325 _ _ _ _]
                  seq-local: [_ w324 _ _ _ _] -> [_ _ w360 _ _ _]
                  tunnel: w322 -> [_ w338 _ w380 w396 w407]
                  frame #0 {
                  }
                  frame #1 {
                    n144 = call "Get_Current_Scan_client.vi"("ADAM Ch Names"=w325) -> ("Numerical Values"=w324:dbl[])  [unwired: 1 in, 2 out]
                    n145 = Index Array(array=w324, index=0) -> (element=w336:dbl)
                    n146 = Index Array(array=w324, index=3) -> (element=w328:dbl)
                    n147 = Index Array(array=w324, index=1) -> (element=w334:dbl)
                    n148 = while {
                      tunnel: w338 -> [w346]
                      tunnel: w336 -> [w345]
                      shift-right: [w345] -> _
                      shift-left: _ -> [w344]
                      shift-right: [w341] -> _
                      shift-left: _ -> [w342]
                      tunnel: w328 -> [w341]
                      tunnel: [w340] -> w327
                      tunnel: [w339] -> w326
                      stop <- TRUE stop-if-true
                      n149 = Not Equal?(x=w345, y=w344) -> (x != y?=w340:bool)
                      n150 = Not Equal?(x=w341, y=w342) -> (x != y?=w339:bool)
                      n151 = case shown="True" w340 {
                        tunnel: w346 -> [_ w347]
                        tunnel: w345 -> [_ w348]
                        frame False {
                        }
                        frame True {
                          n152 = Greater?(x=w348, y=0.2) -> (0:w349:bool)
                          n153 = Boolean To (0,1)(Boolean=w349) -> (0, 1=w352:i16)
                          n154 = dll-call lib="C:/Aerotech/Drivers/OGI_IF.dll" fn="SetFanSystemState"(path in=w347, "Enable"=1, "Fan ONOFF"=w352) -> ()  [unwired: 3 in, 4 out]
                        }
                      }
                    }
                    n155 = Index Array(array=w324, index=2) -> (element=w332:dbl)
                    n156 = Greater?(x=w332, y=0.5) -> (0:w330:bool)
                  }
                  frame #2 {
                    # "allowed temp."
                    n157 = Index Array(array=w360, index=6) -> (element=w358:dbl)
                    n158 = Array Subset(array=w360, index=4, length=3) -> (w362:dbl[])
                    n159 = Array Max & Min(array=w362) -> (max value=w353:dbl)  [unwired: 3 out]
                    n160 = Greater?(x=w358, y=0.5) -> (0:w355:bool)
                    n161 = Greater?(x=w353, y=35.0) -> (0:w356:bool)
                    n162 = And(x=w356, y=w355) -> (x .and. y?=w354:bool)
                    n163 = case shown="True" w354 {
                      tunnel: w353 -> [_ w367]
                      frame False {
                      }
                      frame True {
                        n164 = Format Into String(format string="Aero Tunnel temp is %.1f. The Aero_Tunnel:Fan:Watchdog has therefore been disabled. ", w367) -> (resulting string=w365:string)  [unwired: 2 in, 1 out]
                        n165 = Bundle By Name(cluster=errorcluster {"status"=TRUE, "code"=0, "source"=""} ("error in (no error)"), "source"=w365) -> (w368:errorcluster)
                        n166 = call "EnFlo_Error_Handler.vi"("error in (no error)"=w368, "Error Type"="Aero Tunnel over temp", "Dialog Box (T)"=FALSE) -> ()  [unwired: 3 out]
                        n167 = call "ASYNC_Adam_client.vi"("Values"=dbl[] [0.0, 0.0], "Channel Names"=string[] ["Aero_Tunnel:Fan:Watchdog", "Aero_Tunnel:Road:Watchdog"]) -> ()  [unwired: 1 in, 2 out]
                      }
                    }
                  }
                  frame #3 {
                    n168 = feedback-in #1("Manual Ratio") -> ()
                    n169 = feedback #1() -> (w379:dbl)  [unwired: 1 in]
                    n170 = Not Equal?(x="Manual Ratio", y=w379) -> (x != y?=w375:bool)
                    n171 = Or(x=w375, y=w377) -> (x .or. y?=w376:bool)
                    n172 = case shown="True" w376 {
                      tunnel: w381 -> [_ w389]
                      tunnel: w380 -> [_ w395]
                      tunnel: "Manual Ratio" -> [_ w383]
                      tunnel: "Use Polynomial for Ratio" -> [_ w385]
                      frame False {
                      }
                      frame True {
                        (unwired) dbl[] [0.7807, 0.0283, -0.0013, 2e-05] ("Calib constants")
                        # "no fillets no rolling road no suction"
                        # "rolling road full suction fillets"
                        n173 = call "Polynomial_convert.vi"("Calib constants"=dbl[] [1.1471940648, -0.0162969407, 0.0008616246, -2.02143e-05, 1.764e-07], "Voltage"=w389) -> ("Eng Values"=w384:dbl)  [unwired: 4 in]
                        n174 = Select(t=w384, s=w385, f=w383) -> (s? t:f=w382:dbl)
                        n175 = Equal To 0?(x=w389) -> (x = 0?=w390:bool)
                        n176 = In Range and Coerce(upper limit=1.12, x=w382, lower limit=0.88) -> (coerced(x)=w387:dbl)  [unwired: 1 out]
                        n177 = Select(t=0.88, s=w390, f=w387) -> (s? t:f=w386:dbl)
                        "Required WindSpeedRatio" <- w386
                        n178 = dll-call lib="C:/Aerotech/Drivers/OGI_IF.dll" fn="SetWindSpeedRatio"(path in=w395, "Enable"=1 ("t"), "Required WindSpeedRatio"=w386) -> ()  [unwired: 4 in, 3 out]
                      }
                    }
                  }
                  frame #4 {
                    n179 = while {
                      shift-right: [w399] -> _
                      shift-left: _ -> [w402]
                      tunnel: w397 -> [w399]
                      tunnel: w396 -> [w400]
                      stop <- TRUE stop-if-true
                      n180 = Equal?(x=w399, y=w402) -> (x = y?=w401:bool)
                      n181 = case shown="True" w401 {
                        tunnel: w400 -> [_ w405]
                        tunnel: w399 -> [_ w403]
                        frame False {
                        }
                        frame True {
                          n182 = dll-call lib="C:/Aerotech/Drivers/OGI_IF.dll" fn="SetNewbaroPr_mB"(path in=w405, "Enable"=1, "NewPressure"=w403) -> ()  [unwired: 3 in, 4 out]
                        }
                      }
                    }
                  }
                  frame #5 {
                    n183 = while {
                      shift-right: [w410] -> _
                      shift-left: _ -> [w409]
                      tunnel: w406 -> [w410]
                      tunnel: w407 -> [w412]
                      stop <- TRUE stop-if-true
                      n184 = Compound Arithmetic op=AND(w410, invert w409) -> (w408:bool)
                      n185 = case shown="True" w408 {
                        tunnel: w412 -> [_ w414]
                        frame False {
                        }
                        frame True {
                          n186 = dll-call lib="C:/Aerotech/Drivers/OGI_IF.dll" fn="SetPitotZero"(path in=w414, "Enable"=1) -> ()  [unwired: 2 in, 4 out]
                        }
                      }
                    }
                  }
                }
              }
            }
          }
          frame #12 {
            n187 = while {
              tunnel: w416 -> [w423]
              shift-right: [w421] -> _
              shift-left: _ -> [w420]
              tunnel: w415 -> [w419]
              shift-right: [w417] -> _
              shift-left: _ -> [w418]
              stop <- TRUE stop-if-true
              # "Do every 10 seconds"
              n188 = case shown="True" w419 {
                tunnel: w423 -> [_ _]
                tunnel: [w425 w439] -> w421
                tunnel: w420 -> [w425 w438]
                tunnel: w418 -> [w424 w430]
                tunnel: [w424 w428] -> w417
                frame False {
                  (unwired) FALSE
                }
                frame True {
                  # "Do every 10 minutes"
                  # "flip flop every 10 cycles"
                  n189 = Increment(x=w430) -> (x+1=w427:i32)
                  n190 = Greater?(x=w427, y=60) -> (0:w426:bool)
                  n191 = case shown="False" w426 {
                    tunnel: [w440 0] -> w428
                    tunnel: w427 -> [w440 _]
                    frame False {
                    }
                    frame True {
                    }
                  }
                  n192 = Select(t=1.0, s=w438, f=0.0) -> (s? t:f=w432:dbl)
                  n193 = Bundle By Name(cluster=T6 {"Channel Name"="Aero_Tunnel:Server:Pulse", "New Value"=0.0} ("Update Scan Value Cluster"), "New Value"=w432) -> (w434:T6)
                  n194 = Not(x=w438) -> (.not. x?=w439:bool)
                  n195 = Build Array(w434) -> (w433:T6[])
                  n196 = call "Update_Current_Value_client.vi"("Don't Bother with check?"=TRUE, "Update array in"=w433) -> ()
                }
              }
            }
          }
          frame #13 {
            n197 = while {
              shift-right: [w454] -> _
              shift-left: _ -> [w456]
              tunnel: w442 -> [w455]
              tunnel: w443 -> [w452]
              shift-right: [w450] -> _
              shift-left: _ -> [w451]
              shift-right: [w448] -> _
              shift-left: _ -> [w449]
              shift-right: [w445] -> _
              shift-left: _ -> [w447]
              shift-right: [w444] -> _
              shift-left: _ -> [w446]
              stop <- TRUE stop-if-true
              n198 = stacked-sequence {
                tunnel: w456 -> [w462 _ _ _]
                tunnel: w455 -> [w460 w478 w488 w500]
                tunnel: ["Synch to Wind" _ _ _] -> w454
                tunnel: w452 -> [w457 w476 w486 w502]
                tunnel: w451 -> [_ w475 _ _]
                tunnel: [_ "Start Drive" _ _] -> w450
                tunnel: w449 -> [_ _ w485 _]
                tunnel: [_ _ "Stop drive" _] -> w448
                tunnel: w447 -> [_ _ _ w499]
                tunnel: w446 -> [_ _ _ w496]
                tunnel: [_ _ _ "BL Fan1"] -> w445
                tunnel: [_ _ _ "BL Fan2"] -> w444
                frame #0 {
                  n199 = Not Equal?(x="Synch to Wind", y=w462) -> (x != y?=w461:bool)
                  n200 = Or(x=w461, y=w460) -> (x .or. y?=w458:bool)
                  n201 = case shown="False" w458 {
                    tunnel: "Synch to Wind" -> [_ w471]
                    tunnel: w457 -> [w463 w470]
                    frame False {
                      n202 = Build Array("Aero_Tunnel:Road:Dem_Velocity") -> (w467:string[])
                      n203 = call "Get_Current_Scan_client.vi"("ADAM Ch Names"=w467) -> ("Numerical Values"=w466:dbl[])  [unwired: 1 in, 2 out]
                      n204 = Index Array(array=w466) -> (element=w465:dbl)  [unwired: 1 in]
                      n205 = dll-call lib="C:/Aerotech/Drivers/OGI_IF.dll" fn="SetRoadSpeed_mps"(path in=w463, "Enable"=1, "Required_mps"=w465) -> ()  [unwired: 3 in, 4 out]
                    }
                    frame True {
                      n206 = Boolean To (0,1)(Boolean=w471) -> (0, 1=w472:i16)
                      n207 = To Long Integer(number=w472) -> (32bit integer=w469:i32)
                      n208 = dll-call lib="C:/Aerotech/Drivers/OGI_IF.dll" fn="RoadSyncToWind"(path in=w470, "Enable"=1, "SynchState"=w469) -> ()  [unwired: 3 in, 4 out]
                    }
                  }
                }
                frame #1 {
                  n209 = Not Equal?(x="Start Drive", y=w475) -> (x != y?=w479:bool)
                  n210 = Or(x=w479, y=w478) -> (x .or. y?=w477:bool)
                  n211 = case shown="True" w477 {
                    tunnel: "Start Drive" -> [_ w483]
                    tunnel: w476 -> [_ w481]
                    frame False {
                    }
                    frame True {
                      n212 = Boolean To (0,1)(Boolean=w483) -> (0, 1=w482:i16)
                      n213 = To Long Integer(number=w482) -> (32bit integer=w480:i32)
                      n214 = dll-call lib="C:/Aerotech/Drivers/OGI_IF.dll" fn="StartRoadDrive"(path in=w481, "Enable"=w480) -> ()  [unwired: 2 in, 4 out]
                    }
                  }
                }
                frame #2 {
                  n215 = Not Equal?(x="Stop drive", y=w485) -> (x != y?=w489:bool)
                  n216 = Or(x=w489, y=w488) -> (x .or. y?=w487:bool)
                  n217 = case shown="True" w487 {
                    tunnel: "Stop drive" -> [_ w493]
                    tunnel: w486 -> [_ w491]
                    frame False {
                    }
                    frame True {
                      n218 = Boolean To (0,1)(Boolean=w493) -> (0, 1=w492:i16)
                      n219 = To Long Integer(number=w492) -> (32bit integer=w490:i32)
                      n220 = dll-call lib="C:/Aerotech/Drivers/OGI_IF.dll" fn="RoadStop"(path in=w491, "Enable"=w490) -> ()  [unwired: 2 in, 4 out]
                    }
                  }
                }
                frame #3 {
                  n221 = Not Equal?(x=w496, y="BL Fan2") -> (x != y?=w497:bool)
                  n222 = Not Equal?(x="BL Fan1", y=w499) -> (x != y?=w498:bool)
                  n223 = Compound Arithmetic op=OR(w498, w497, w500) -> (w501:bool)
                  n224 = case shown="True" w501 {
                    tunnel: w502 -> [_ w504]
                    tunnel: "BL Fan1" -> [_ w506]
                    tunnel: "BL Fan2" -> [_ w505]
                    frame False {
                    }
                    frame True {
                      w503 = 1 ("BL Fan (1 or 2)")
                      n225 = dll-call lib="C:/Aerotech/Drivers/OGI_IF.dll" fn="SetBoundaryPerc"(path in=w504, "enable"=w503, "BL Fan (1 or 2)"=1, "New Percentage"=w506) -> ()  [unwired: 4 in, 4 out]
                      n226 = dll-call lib="C:/Aerotech/Drivers/OGI_IF.dll" fn="SetBoundaryPerc"(path in=w504, "enable"=w503, "BL Fan (1 or 2)"=2, "New Percentage"=w505) -> ()  [unwired: 4 in, 4 out]
                    }
                  }
                }
              }
            }
          }
        }
        n227 = case shown="True" w20 {
          tunnel: [w46 w53] -> w36
          tunnel: w35 -> [_ w52]
          tunnel: w34 -> [w46 w51]
          tunnel: w33 -> [_ w50]
          tunnel: w21 -> [_ w47]
          frame False {
          }
          frame True {
            w48 = FALSE  # Give Variance
            w49 = 1.0  # Averaging Period (s)
            n228 = call "Upload_To_ADAM_Server.vi"("First Loop"=w47, "Averaging Period (s)"=w49, "Shift In"=w51, "Channel Values"=w52, "Give Variance"=w48, "Channel Names"=w50) -> ("Shift Out"=w53:dbl[])
          }
        }
        n229 = node-c288() -> ()  [unwired: 1 in, 1 out]
      }
      n230 = node-c288(w15) -> ()  [unwired: 1 out]
    }
    frame #3 {
      n231 = dll-call lib="C:/Aerotech/Drivers/OGI_IF.dll" fn="CloseLink"(path in=w513) -> ()  [unwired: 2 in, 3 out]
    }
  }
